vi "Select Tovey Data.vi"(8 "error in (no error)":errorcluster, 9 "End Time":dbl, 10 "Start Time":dbl, 11 "Model in":refnum<class "Model.lvclass">) -> (0 "error out":errorcluster, 1 "StartIndex":i32, 2 "Data":T1[](array[typedef]) {"Timestamp" format="%.4f"; "Mz" format="%.4f"; "My" format="%.4f"; "Mx" format="%.4f"; "Fz" format="%.4f"; "Fy" format="%.4f"; "Fx" format="%.4f"}, 3 "Model out":refnum<class "Model.lvclass">)   [LabVIEW 2016]
uses:
  Typedefs/ToveyEngData.ctl
  Model.lvclass
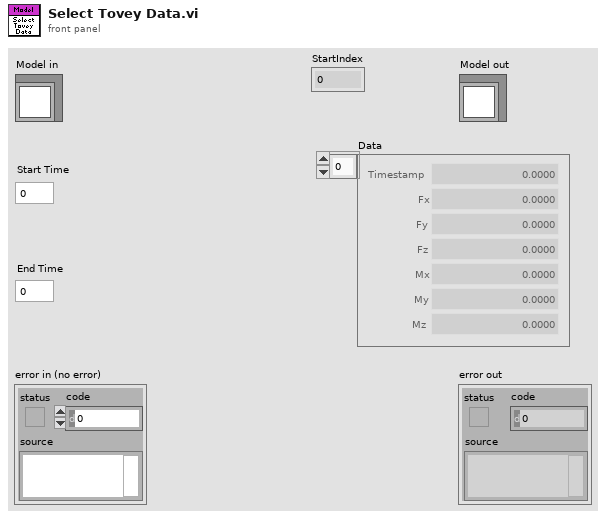
[diagram p1: front panel]
types:
  T1 = typedef "ToveyEngData.ctl" = cluster{"Timestamp":dbl, "Fx":dbl, "Fy":dbl, "Fz":dbl, "Mx":dbl, "My":dbl, "Mz":dbl}
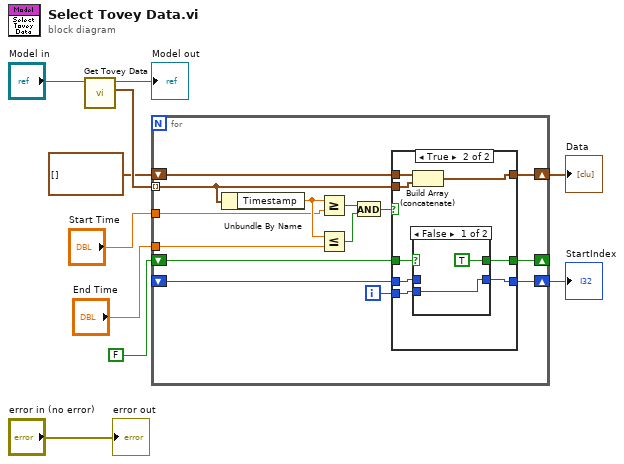
[diagram p0: block diagram]
diagram:
  n1 = call "Get Tovey Data.vi"("Model in"="Model in") -> ("ToveyData"=w9:T1[], "Model out"=→"Model out":refnum<class "Model.lvclass">)  [unwired: 9 in]
  n2 = for {
    tunnel: w9 -> [w20] mode=indexing
    shift-right: [w19] -> w5
    shift-left: T1[] [] -> [w18]
    tunnel: "Start Time" -> [w17]
    tunnel: "End Time" -> [w16]
    shift-right: [w14] -> _
    shift-left: FALSE -> [w15]
    shift-right: [w13] -> w1
    shift-left: _ -> [w11]
    i -> [w12]
    n3 = Unbundle By Name(w20) -> ("Timestamp"=w24:dbl)
    n4 = Greater Or Equal?(x=w24, y=w17) -> (x >= y?=w23:bool)
    n5 = Less Or Equal?(x=w24, y=w16) -> (x <= y?=w22:bool)
    n6 = And(x=w23, y=w22) -> (x .and. y?=w21:bool)
    n7 = case shown="True" w21 {
      tunnel: w20 -> [_ w35]
      tunnel: [w27 w34] -> w19
      tunnel: w18 -> [w27 w33]
      tunnel: w15 -> [w26 w32]
      tunnel: [w26 w31] -> w14
      tunnel: [w25 w30] -> w13
      tunnel: w12 -> [_ w29]
      tunnel: w11 -> [w25 w28]
      frame False {
      }
      frame True {
        n8 = Build Array (concatenate)(w33, w35) -> (w34:T1[])
        n9 = case shown="False" w32 {
          selector: w32 -> [_ w39]
          tunnel: [TRUE w39] -> w31
          tunnel: [w36 w38] -> w30
          tunnel: w29 -> [w36 _]
          tunnel: w28 -> [_ w38]
          frame False {
          }
          frame True {
          }
        }
      }
    }
  }
  "Data" <- w5
  "StartIndex" <- w1
  "error out" <- "error in (no error)"
